vi "Search_1D_Array(DBL).vi"(0 "Array":dbl[](array[numeric]), 2 "Element Data":dbl, 3 "Start Index (0)":i32) -> (7 "Indicies of Elements":i32[](array[numeric]), 9 "Elements":dbl[](array[numeric]))   [LabVIEW 2011]
doc: "Searches for all element data matches in array"
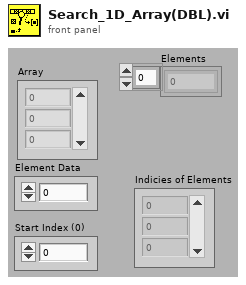
[diagram p1: front panel]
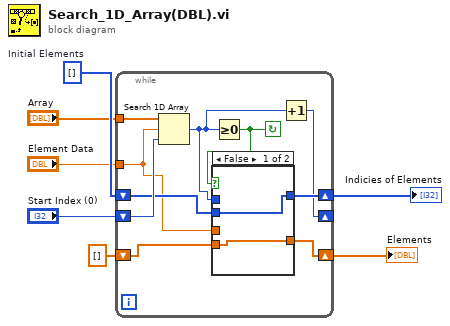
[diagram p0: block diagram]
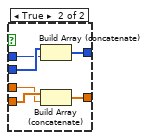
[diagram p2: hidden frame]
diagram:
  w7 = i32[] []  # Initial Elements
  n1 = while {
    shift-right: [w13] -> _
    shift-left: "Start Index (0)" -> [w17]
    shift-right: [w14] -> w3
    shift-left: w7 -> [w15]
    tunnel: "Array" -> [w16]
    tunnel: "Element Data" -> [w8]
    shift-right: [w11] -> w2
    shift-left: dbl[] [] -> [w12]
    stop <- w10 continue-if-true
    n2 = Search 1D Array(1D array=w16, element=w8, start index (0)=w17) -> (index of element=w9:i32)
    n3 = Greater Or Equal To 0?(x=w9) -> (x >= 0?=w10:bool)
    n4 = case shown="False" w10 {
      tunnel: w15 -> [w19 w25]
      tunnel: [w19 w24] -> w14
      tunnel: w12 -> [w18 w22]
      tunnel: [w18 w23] -> w11
      tunnel: w9 -> [_ w21]
      tunnel: w8 -> [_ w20]
      frame False {
      }
      frame True {
        n5 = Build Array (concatenate)(w25, w21) -> (w24:i32[])
        n6 = Build Array (concatenate)(w22, w20) -> (w23:dbl[])
      }
    }
    n7 = Increment(x=w9) -> (x+1=w13:i32)
  }
  "Indicies of Elements" <- w3
  "Elements" <- w2
